vi "EPTxRTmul-inj_Timing1.0.vi"(3 "Control_Config_in":T13={"RT_Input"={"Load"=FALSE, "History_[CAD]"=63, "Stall_Speed_[RPM]"=200.0, "Delay_time[ms]"=0.0}, " PatternConfig"={"Aux_Offset_1_[CAD]"=0.0, "Aux_Offset_2_[CAD]"=0.0, "Aux_Offset_3_[CAD]"=0.0, "Aux_Offset_4_[CAD]"=0.0, "Max_Rate_[Hz]"=0.0}, "SimulatorConfig"={"Sim_Speed_[RPM]"=1000.0, "Ramp_Rate"=50.0, "Rotations"=2, "Pause"=FALSE, "Pause_Angle_[CAD]"=0.0, "Max_Offset_[RPM]"=0.0, "Cylinders"=6}, "EPTxState"={"Sync_Enable"=TRUE, "Clear_Errors"=FALSE, "Sim_Enable"=FALSE, "Sim_Speed_[RPM]"=1000.0}, "EPTxFilters"={"Primary_[s]"=5e-06, "Aux_1_[s]"=5e-06, "Aux_2_[s]"=0.0, "Aux_3_[s]"=0.0, "Aux_4_[s]"=0.0}, "EPTxSupervisor_rt"={"Sync"=FALSE, "CurrentCAD"=0.0, "MaxCAD"=720.0, "HistoryCAD"=61.0, "CADRate"=0.0, "AvgSpeed"=0.0, "Config"=FALSE, "Rcvg_Primary"=FALSE, "Stall"=FALSE, "Overflow"=FALSE, "Ratio_Error"=FALSE, "Pattern_Error"=FALSE, "Aux_Warning"=FALSE, "Watchdog_Error"=FALSE}, "Control_strategy_input"={"Injection_DBTDC"=6.0, "Injection_duration[ms]"=2.0}} caption="簇" {"EPTxFilters"."Aux_4_[s]" format="%#_6p"; "EPTxFilters"."Aux_3_[s]" format="%#_6p"; "EPTxFilters"."Aux_2_[s]" format="%#_6p"; "EPTxFilters"."Aux_1_[s]" format="%#_6p"; "EPTxFilters"."Primary_[s]" format="%#_6p"; "PatternConfig"."Max_Rate_[Hz]" format="%#_3p"}) -> (0 "Control_Config_out":T7={"Config_number"={"EPTxConfig"=0, "EPTxSimulatorConfig"=0}, "Lighting"={"Pattern_Loading"=FALSE, "Sim_Loading"=FALSE, "Config_Loading"=FALSE}, "CylinderSig"={"CylinderSig_1"={"Cylinder1_H_R[CAD]"=204.0, "Cylinder1_H_F[CAD]"=210.0}, "CylinderSig_2"={"Cylinder2_H_R[CAD]"=684.0, "Cylinder2_H_F[CAD]"=690.0}, "CylinderSig_3"={"Cylinder3_H_R[CAD]"=444.0, "Cylinder3_H_F[CAD]"=450.0}, "CylinderSig_4"={"Cylinder4_H_R[CAD]"=90.0, "Cylinder4_H_F[CAD]"=100.0}, "CylinderSig_5"={"Cylinder5_H_R[CAD]"=324.0, "Cylinder5_H_F[CAD]"=330.0}, "CylinderSig_6"={"Cylinder6_H_R[CAD]"=0.0, "Cylinder6_H_F[CAD]"=0.0}}, "EPTxPatternConfig"={"Address"=0.0, "Pattern"={"Primary"=0.0, "Primary_State"=FALSE, "Aux_1"=0.0, "Aux_1_State"=FALSE, "Aux_2"=0.0, "Aux_2_State"=FALSE, "Aux_3"=0.0, "Aux_3_State"=FALSE, "Aux_4"=0.0, "Aux_4_State"=FALSE}}, "EPTxControl"={"Sync_Enable"=FALSE, "Clear_Errors"=FALSE, "Sim_Enable"=FALSE, "Sim_Rate"=63.999996185302734, "Watchdog"=FALSE}, "Tick_output"={"Duration[Ticks]"=0, "Delay[Ticks]"=0}, "EPTxData"={"Sync"=TRUE, "CurrentCAD"=122.91406, "Speed_[RPM]"=999.75, "Config"=FALSE, "Rcvg_Primary"=TRUE, "Stall"=FALSE, "Overflow"=FALSE, "Ratio_Error"=FALSE, "Pattern_Error"=FALSE, "Aux_Warning"=FALSE, "Watchdog_Error"=FALSE}} caption="簇" {"EPTxPatternConfig"."Pattern"."Aux_4" format="%#_16g"; "EPTxPatternConfig"."Pattern"."Aux_3" format="%#_16g"; "EPTxPatternConfig"."Pattern"."Aux_2" format="%#_16g"; "EPTxPatternConfig"."Pattern"."Aux_1" format="%#_16g"; "EPTxPatternConfig"."Pattern"."Primary" format="%#_16g"})   [LabVIEW 2020]
uses:
  <vilib>/Powertrain Controls/Device Drivers/Engine Position Tracking/EPTx/RevA/RT/Controls/Pattern Config.ctl
  <vilib>/Powertrain Controls/Device Drivers/Engine Position Tracking/EPTx/RevA/RT/Controls/Simulator Config.ctl
  <vilib>/Powertrain Controls/Device Drivers/Engine Position Tracking/EPTx/RevA/RT/Controls/EPTxState.ctl
  <vilib>/Powertrain Controls/Device Drivers/Engine Position Tracking/EPTx/RevA/RT/Controls/EPTxFilters.ctl
  <vilib>/Powertrain Controls/Device Drivers/Engine Position Tracking/EPTx/RevA/FPGA/Controls/EPTxSupervisor.ctl
  <vilib>/Powertrain Controls/Device Drivers/Engine Position Tracking/EPTx/RevA/FPGA/Controls/EPTxConfig.ctl
  <vilib>/Powertrain Controls/Device Drivers/Engine Position Tracking/EPTx/RevA/FPGA/Controls/EPTxSimulatorConfig.ctl
  <vilib>/Powertrain Controls/Device Drivers/Engine Position Tracking/EPTx/RevA/FPGA/Controls/EPTxPatternConfig.ctl
  <vilib>/Powertrain Controls/Device Drivers/Engine Position Tracking/EPTx/RevA/FPGA/Controls/Patterns.ctl
  <vilib>/Powertrain Controls/Device Drivers/Engine Position Tracking/EPTx/RevA/FPGA/Controls/EPTxControl.ctl
  <vilib>/Powertrain Controls/Device Drivers/Engine Position Tracking/EPTx/RevA/RT/Controls/EPTxData.ctl
  <vilib>/Powertrain Controls/Device Drivers/Engine Position Tracking/EPTx/RevA/RT/Controls/EPTxPattern.ctl
  <vilib>/Powertrain Controls/Device Drivers/Engine Position Tracking/EPTx/RevA/RT/Controls/Pattern.ctl
  <vilib>/Powertrain Controls/Device Drivers/Engine Position Tracking/EPTx/RevA/RT/Controls/EPTxSettings.ctl
  <vilib>/Powertrain Controls/Device Drivers/Engine Position Tracking/EPTx/RevA/RT/Controls/Settings - Tooth.ctl
  <vilib>/Powertrain Controls/Device Drivers/Engine Position Tracking/EPTx/RevA/RT/Controls/Direction Detection.ctl
  <vilib>/Powertrain Controls/Device Drivers/Engine Position Tracking/EPTx/RevA/RT/Controls/Settings - Pattern.ctl
  <vilib>/Powertrain Controls/Device Drivers/Engine Position Tracking/EPTx/RevA/RT/Controls/Settings - Token.ctl
  <vilib>/Powertrain Controls/Device Drivers/Engine Position Tracking/EPTx/RevA/RT/Controls/Aux Signal.ctl
  <vilib>/Powertrain Controls/Device Drivers/Engine Position Tracking/EPTx/RevA/RT/Controls/Aux Type.ctl
  <vilib>/Powertrain Controls/Device Drivers/Engine Position Tracking/EPTx/RevA/RT/Controls/Aux Threshold.ctl
  <vilib>/Powertrain Controls/Device Drivers/Engine Position Tracking/EPTx/RevA/RT/EPTx - RevA - RT.lvlib
  <vilib>/Powertrain Controls/Device Drivers/Engine Position Tracking/EPTx/RevA/FPGA/EPTx - RevA - FPGA.lvlib
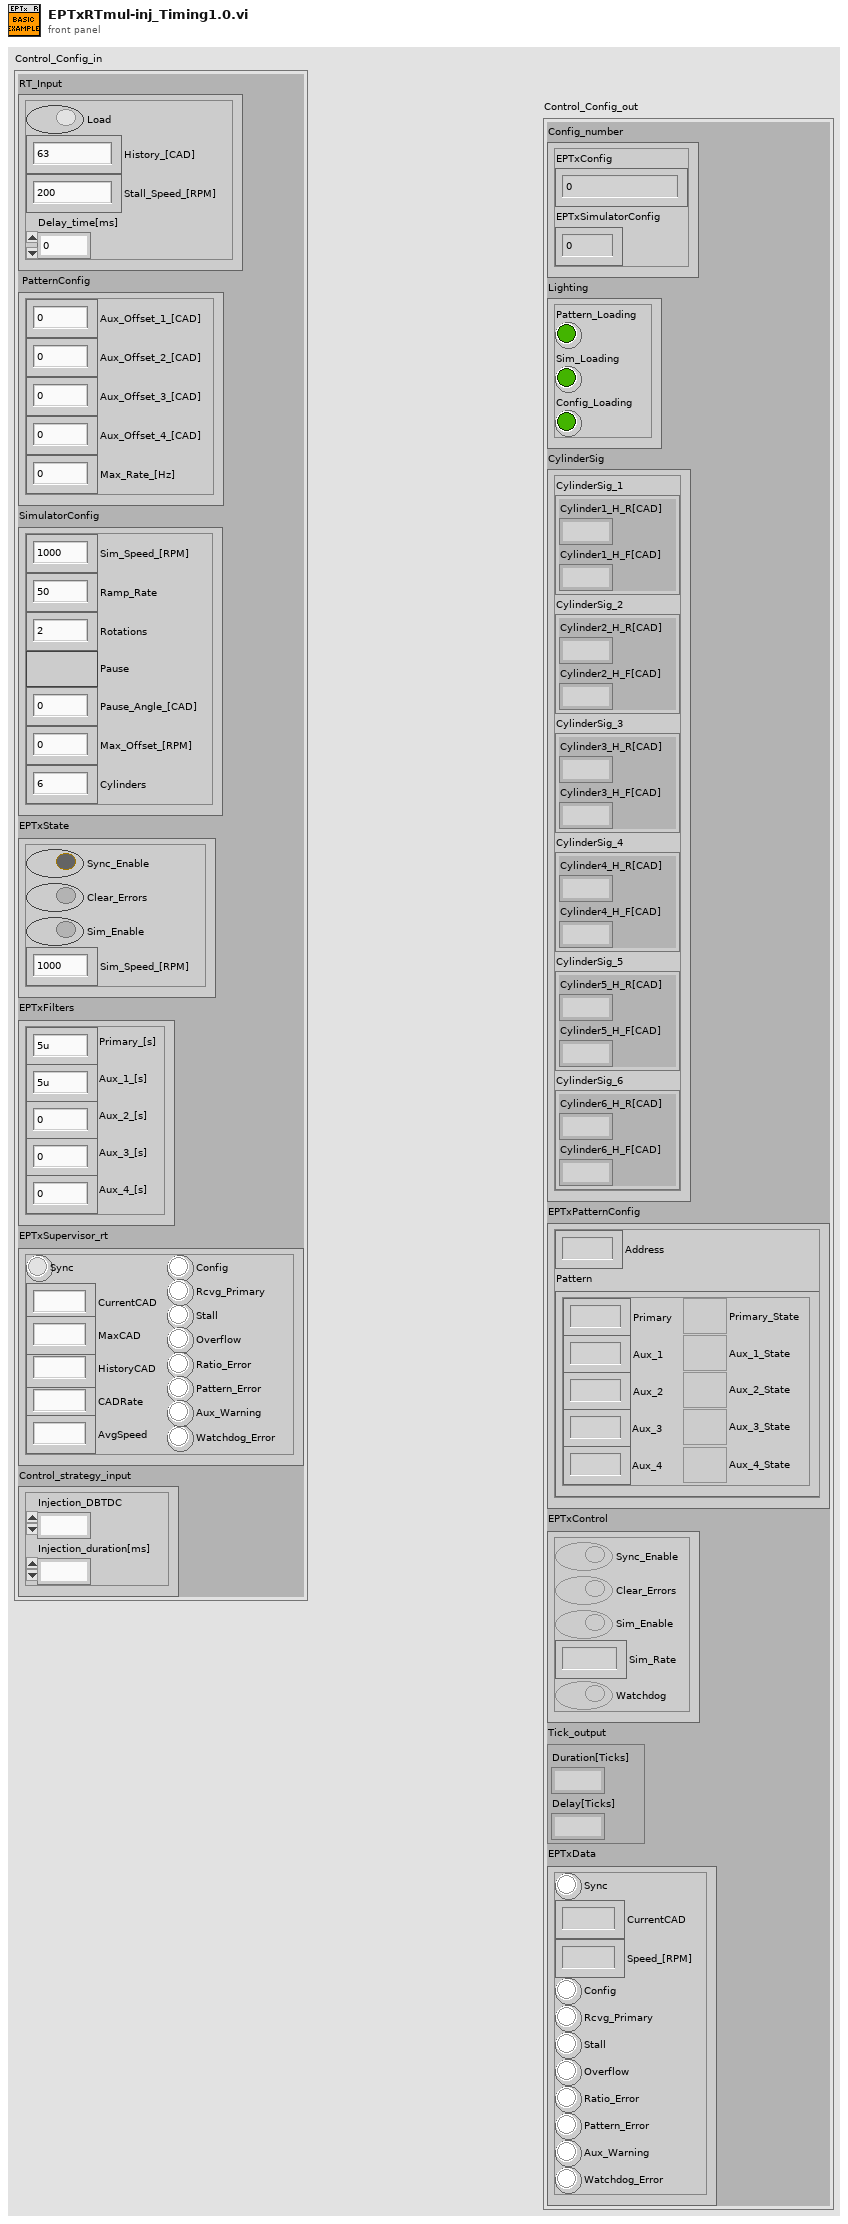
[diagram p1: front panel]
types:
  T1 = typedef "EPTx - RevA - FPGA.lvlib/EPTxConfig.ctl" = u64
  T2 = typedef "EPTx - RevA - FPGA.lvlib/EPTxSimulatorConfig.ctl" = u32
  T3 = typedef "EPTx - RevA - FPGA.lvlib/EPTxPatternConfig.ctl" = cluster{"Address":fxp<+,14,14>, "Pattern":T4}
  T4 = typedef "EPTx - RevA - FPGA.lvlib/Patterns.ctl" = cluster{"Primary":fxp<+,19,12>, "Primary_State":bool, "Aux_1":fxp<+,19,12>, "Aux_1_State":bool, "Aux_2":fxp<+,19,12>, "Aux_2_State":bool, "Aux_3":fxp<+,19,12>, "Aux_3_State":bool, "Aux_4":fxp<+,19,12>, "Aux_4_State":bool}
  T5 = typedef "EPTx - RevA - FPGA.lvlib/EPTxControl.ctl" = cluster{"Sync_Enable":bool, "Clear_Errors":bool, "Sim_Enable":bool, "Sim_Rate":fxp<+,24,6>, "Watchdog":bool}
  T6 = typedef "EPTx - RevA - RT.lvlib/EPTxData.ctl" = cluster{"Sync":bool, "CurrentCAD":sgl, "Speed_[RPM]":sgl, "Config":bool, "Rcvg_Primary":bool, "Stall":bool, "Overflow":bool, "Ratio_Error":bool, "Pattern_Error":bool, "Aux_Warning":bool, "Watchdog_Error":bool}
  T7 = cluster{"Config_number":cluster{"EPTxConfig":T1, "EPTxSimulatorConfig":T2}, "Lighting":cluster{"Pattern_Loading":bool, "Sim_Loading":bool, "Config_Loading":bool}, "CylinderSig":cluster{"CylinderSig_1":cluster{"Cylinder1_H_R[CAD]":fxp<+,18,11>, "Cylinder1_H_F[CAD]":fxp<+,18,11>}, "CylinderSig_2":cluster{"Cylinder2_H_R[CAD]":fxp<+,18,11>, "Cylinder2_H_F[CAD]":fxp<+,18,11>}, "CylinderSig_3":cluster{"Cylinder3_H_R[CAD]":fxp<+,18,11>, "Cylinder3_H_F[CAD]":fxp<+,18,11>}, "CylinderSig_4":cluster{"Cylinder4_H_R[CAD]":fxp<+,18,11>, "Cylinder4_H_F[CAD]":fxp<+,18,11>}, "CylinderSig_5":cluster{"Cylinder5_H_R[CAD]":fxp<+,18,11>, "Cylinder5_H_F[CAD]":fxp<+,18,11>}, "CylinderSig_6":cluster{"Cylinder6_H_R[CAD]":fxp<+,18,11>, "Cylinder6_H_F[CAD]":fxp<+,18,11>}}, "EPTxPatternConfig":T3, "EPTxControl":T5, "Tick_output":cluster{"Duration[Ticks]":u16, "Delay[Ticks]":u16}, "EPTxData":T6}
  T8 = typedef "EPTx - RevA - RT.lvlib/Pattern Config.ctl" = cluster{"Aux_Offset_1_[CAD]":sgl, "Aux_Offset_2_[CAD]":sgl, "Aux_Offset_3_[CAD]":sgl, "Aux_Offset_4_[CAD]":sgl, "Max_Rate_[Hz]":sgl}
  T9 = typedef "EPTx - RevA - RT.lvlib/Simulator Config.ctl" = cluster{"Sim_Speed_[RPM]":sgl, "Ramp_Rate":sgl, "Rotations":u8, "Pause":bool, "Pause_Angle_[CAD]":sgl, "Max_Offset_[RPM]":sgl, "Cylinders":u8}
  T10 = typedef "EPTx - RevA - RT.lvlib/EPTxState.ctl" = cluster{"Sync_Enable":bool, "Clear_Errors":bool, "Sim_Enable":bool, "Sim_Speed_[RPM]":sgl}
  T11 = typedef "EPTx - RevA - RT.lvlib/EPTxFilters.ctl" = cluster{"Primary_[s]":sgl, "Aux_1_[s]":sgl, "Aux_2_[s]":sgl, "Aux_3_[s]":sgl, "Aux_4_[s]":sgl}
  T12 = typedef "EPTx - RevA - FPGA.lvlib/EPTxSupervisor.ctl" = cluster{"Sync":bool, "CurrentCAD":fxp<+,18,11>, "MaxCAD":fxp<+,11,11>, "HistoryCAD":fxp<+,11,11>, "CADRate":fxp<+,22,8>, "AvgSpeed":fxp<+,17,15>, "Config":bool, "Rcvg_Primary":bool, "Stall":bool, "Overflow":bool, "Ratio_Error":bool, "Pattern_Error":bool, "Aux_Warning":bool, "Watchdog_Error":bool}
  T13 = cluster{"RT_Input":cluster{"Load":bool, "History_[CAD]":u8, "Stall_Speed_[RPM]":sgl, "Delay_time[ms]":sgl}, " PatternConfig":T8, "SimulatorConfig":T9, "EPTxState":T10, "EPTxFilters":T11, "EPTxSupervisor_rt":T12, "Control_strategy_input":cluster{"Injection_DBTDC":sgl, "Injection_duration[ms]":sgl}}
  T14 = cluster{"Duration[Ticks]":u16, "Delay[Ticks]":u16}
  T15 = cluster{"CylinderSig_1":cluster{"Cylinder1_H_R [CAD]":fxp<+,18,11>, "Cylinder1_H_F [CAD]":fxp<+,18,11>}, "CylinderSig_2":cluster{"Cylinder2_H_R [CAD]":fxp<+,18,11>, "Cylinder2_H_F [CAD]":fxp<+,18,11>}, "CylinderSig_3":cluster{"Cylinder3_H_R [CAD]":fxp<+,18,11>, "Cylinder3_H_F [CAD]":fxp<+,18,11>}, "CylinderSig_4":cluster{"Cylinder4_H_R [CAD]":fxp<+,18,11>, "Cylinder4_H_F [CAD]":fxp<+,18,11>}, "CylinderSig_5":cluster{"Cylinder5_H_R [CAD]":fxp<+,18,11>, "Cylinder5_H_F [CAD]":fxp<+,18,11>}, "CylinderSig_6":cluster{"Cylinder6_H_R [CAD]":fxp<+,18,11>, "Cylinder6_H_F [CAD]":fxp<+,18,11>}}
  T16 = cluster{"Cylinder6_H_R [CAD]":fxp<+,18,11>, "Cylinder6_H_F [CAD]":fxp<+,18,11>}
  T17 = cluster{"Cylinder5_H_R [CAD]":fxp<+,18,11>, "Cylinder5_H_F [CAD]":fxp<+,18,11>}
  T18 = cluster{"Cylinder4_H_R [CAD]":fxp<+,18,11>, "Cylinder4_H_F [CAD]":fxp<+,18,11>}
  T19 = cluster{"Cylinder3_H_R [CAD]":fxp<+,18,11>, "Cylinder3_H_F [CAD]":fxp<+,18,11>}
  T20 = cluster{"Cylinder2_H_R [CAD]":fxp<+,18,11>, "Cylinder2_H_F [CAD]":fxp<+,18,11>}
  T21 = cluster{"Cylinder1_H_R [CAD]":fxp<+,18,11>, "Cylinder1_H_F [CAD]":fxp<+,18,11>}
  T22 = cluster{"EPTxConfig":T1, "EPTxSimulatorConfig":T2}
  T23 = cluster{"Pattern Loading":bool, "Sim Loading":bool, "Config Loading":bool}
  T24 = cluster{"Load":bool, "History_[CAD]":u8, "Stall_Speed_[RPM]":sgl, "Delay_time[ms]":sgl}
  T25 = cluster{"Injection_DBTDC":sgl, "Injection_duration[ms]":sgl}
  T26 = typedef "EPTx - RevA - RT.lvlib/EPTxSettings.ctl" = cluster{"Rotation":u8, "Ratios":sgl[], "Thresholds":sgl[], "Tooth":T27, "Pattern":T29[], "Token":T30[], "Aux Threshold Min":T33, "Aux Threshold Max":T33}
  T27 = typedef "EPTx - RevA - RT.lvlib/Settings - Tooth.ctl" = cluster{"Rising Edge":bool, "Falling Edge":bool, "Direction\nDetection":T28, "Level":bool, "Parameter":sgl}
  T28 = typedef "EPTx - RevA - RT.lvlib/Direction Detection.ctl" = enum16{"None", "Aux Signal", "Length"}
  T29 = typedef "EPTx - RevA - RT.lvlib/Settings - Pattern.ctl" = cluster{"Ratio Index":u8, "Ratio Count":u16, "Angle":sgl, "dAngle":sgl}
  T30 = typedef "EPTx - RevA - RT.lvlib/Settings - Token.ctl" = cluster{"Length":u16, "Start Index":u8, "Start Count":u16, "Aux 1":T31, "Aux 1 Type":T32, "Aux 1 Max":u16, "Aux 1 Min":u16, "Aux 2":T31, "Aux 2 Type":T32, "Aux 2 Max":u16, "Aux 2 Min":u16, "End Index":u8, "End Count":u16}
  T31 = typedef "EPTx - RevA - RT.lvlib/Aux Signal.ctl" = enum8{"---", "Aux 1", "Aux 2", "Aux 3", "Aux 4"}
  T32 = typedef "EPTx - RevA - RT.lvlib/Aux Type.ctl" = enum8{"Falling", "Rising", "Low", "High", "Ratio"}
  T33 = typedef "EPTx - RevA - RT.lvlib/Aux Threshold.ctl" = cluster{"Aux 1":sgl, "Aux 2":sgl, "Aux 3":sgl, "Aux 4":sgl}
  T34 = typedef "EPTx - RevA - RT.lvlib/EPTxPattern.ctl" = cluster{"Rotations":u8, "Cylinders":u8, "Primary":T35[], "Aux 1":T35[], "Aux 2":T35[], "Aux 3":T35[], "Aux 4":T35[]}
  T35 = typedef "EPTx - RevA - RT.lvlib/Pattern.ctl" = cluster{"Angle":sgl, "State":bool}
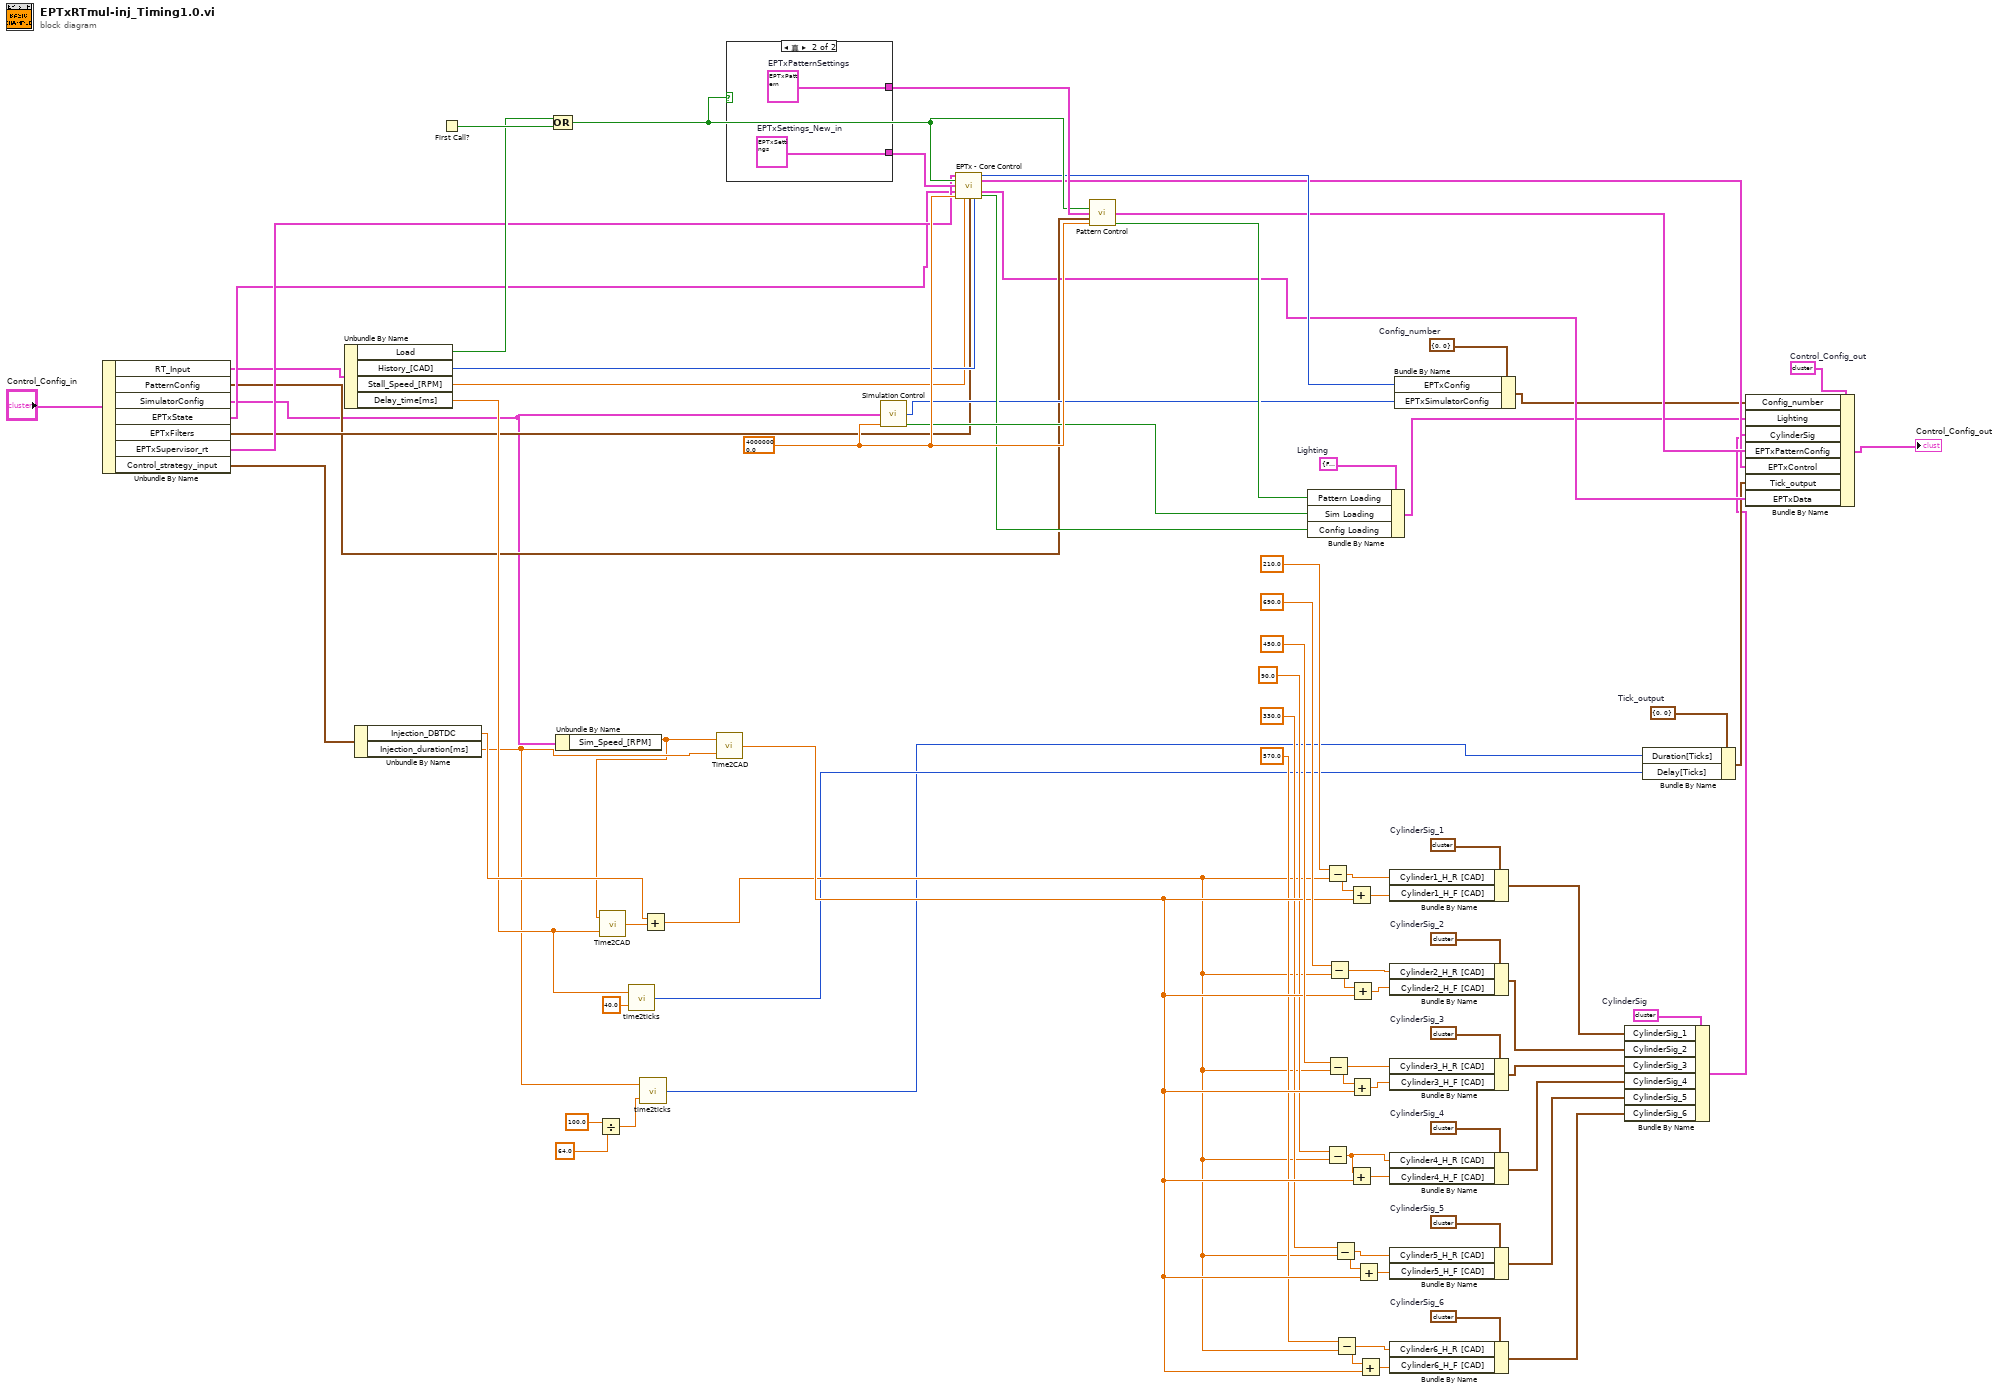
[diagram p0: block diagram]
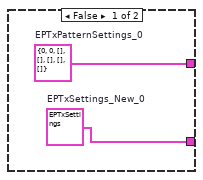
[diagram p2: hidden frame]
diagram:
  w10 = T7 {"Config_number"={"EPTxConfig"=0, "EPTxSimulatorConfig"=0}, "Lighting"={"Pattern_Loading"=FALSE, "Sim_Loading"=FALSE, "Config_Loading"=FALSE}, "CylinderSig"={"CylinderSig_1"={"Cylinder1_H_R[CAD]"=204.0, "Cylinder1_H_F[CAD]"=210.0}, "CylinderSig_2"={"Cylinder2_H_R[CAD]"=684.0, "Cylinder2_H_F[CAD]"=690.0}, "CylinderSig_3"={"Cylinder3_H_R[CAD]"=444.0, "Cylinder3_H_F[CAD]"=450.0}, "CylinderSig_4"={"Cylinder4_H_R[CAD]"=90.0, "Cylinder4_H_F[CAD]"=100.0}, "CylinderSig_5"={"Cylinder5_H_R[CAD]"=324.0, "Cylinder5_H_F[CAD]"=330.0}, "CylinderSig_6"={"Cylinder6_H_R[CAD]"=0.0, "Cylinder6_H_F[CAD]"=0.0}}, "EPTxPatternConfig"={"Address"=0.0, "Pattern"={"Primary"=0.0, "Primary_State"=FALSE, "Aux_1"=0.0, "Aux_1_State"=FALSE, "Aux_2"=0.0, "Aux_2_State"=FALSE, "Aux_3"=0.0, "Aux_3_State"=FALSE, "Aux_4"=0.0, "Aux_4_State"=FALSE}}, "EPTxControl"={"Sync_Enable"=FALSE, "Clear_Errors"=FALSE, "Sim_Enable"=FALSE, "Sim_Rate"=63.999996185302734, "Watchdog"=FALSE}, "Tick_output"={"Duration[Ticks]"=0, "Delay[Ticks]"=0}, "EPTxData"={"Sync"=TRUE, "CurrentCAD"=122.91406, "Speed_[RPM]"=999.75, "Config"=FALSE, "Rcvg_Primary"=TRUE, "Stall"=FALSE, "Overflow"=FALSE, "Ratio_Error"=FALSE, "Pattern_Error"=FALSE, "Aux_Warning"=FALSE, "Watchdog_Error"=FALSE}}  # Control_Config_out
  w25 = T14 {"Duration[Ticks]"=0, "Delay[Ticks]"=0}  # Tick_output
  w41 = T15 {"CylinderSig_1"={"Cylinder1_H_R [CAD]"=204.0, "Cylinder1_H_F [CAD]"=210.0}, "CylinderSig_2"={"Cylinder2_H_R [CAD]"=684.0, "Cylinder2_H_F [CAD]"=690.0}, "CylinderSig_3"={"Cylinder3_H_R [CAD]"=444.0, "Cylinder3_H_F [CAD]"=450.0}, "CylinderSig_4"={"Cylinder4_H_R [CAD]"=90.0, "Cylinder4_H_F [CAD]"=100.0}, "CylinderSig_5"={"Cylinder5_H_R [CAD]"=324.0, "Cylinder5_H_F [CAD]"=330.0}, "CylinderSig_6"={"Cylinder6_H_R [CAD]"=0.0, "Cylinder6_H_F [CAD]"=0.0}}  # CylinderSig
  w58 = T16 {"Cylinder6_H_R [CAD]"=0.0, "Cylinder6_H_F [CAD]"=0.0}  # CylinderSig_6
  w59 = T17 {"Cylinder5_H_R [CAD]"=324.0, "Cylinder5_H_F [CAD]"=330.0}  # CylinderSig_5
  w60 = T18 {"Cylinder4_H_R [CAD]"=90.0, "Cylinder4_H_F [CAD]"=100.0}  # CylinderSig_4
  w61 = T19 {"Cylinder3_H_R [CAD]"=444.0, "Cylinder3_H_F [CAD]"=450.0}  # CylinderSig_3
  w62 = T20 {"Cylinder2_H_R [CAD]"=684.0, "Cylinder2_H_F [CAD]"=690.0}  # CylinderSig_2
  w63 = T21 {"Cylinder1_H_R [CAD]"=204.0, "Cylinder1_H_F [CAD]"=210.0}  # CylinderSig_1
  w69 = T22 {"EPTxConfig"=0, "EPTxSimulatorConfig"=0}  # Config_number
  w73 = T23 {"Pattern Loading"=FALSE, "Sim Loading"=FALSE, "Config Loading"=FALSE}  # Lighting
  w77 = sgl 40000000.0 ("Frequency (40M) [Hz]")
  n1 = Unbundle By Name("Control_Config_in") -> ("RT_Input"=w14:T24, "PatternConfig"=w13:T8, "SimulatorConfig"=w12:T9, "EPTxState"=w16:T10, "EPTxFilters"=w15:T11, "EPTxSupervisor_rt"=w17:T12, "Control_strategy_input"=w11:T25)
  n2 = Unbundle By Name(w14) -> ("Load"=w66:bool, "History_[CAD]"=w65:u8, "Stall_Speed_[RPM]"=w64:sgl, "Delay_time[ms]"=w27:sgl)
  n3 = Unbundle By Name(w11) -> ("Injection_DBTDC"=w30:sgl, "Injection_duration[ms]"=w26:sgl)
  n4 = First Call?() -> (First Call?: T/F=w75:bool)
  n5 = Compound Arithmetic op=OR ("复合运算")(w66, w75) -> (w74:bool)
  n6 = Unbundle By Name(w12) -> ("Sim_Speed_[RPM]"=w1:sgl)
  n7 = Divide(x=100.0, y=64.0) -> (x/y=w19:dbl)
  n8 = call <vilib>:"Time2CAD.vi"("Time [ms]"=w27, "Speed (RPM)"=w1) -> ("CAD"=w28:sgl)
  n9 = call <vilib>:"time2ticks.vi"("Clock Frequency (MHz, 40)"=sgl 40.0, "Time (msec)"=w27) -> ("Ticks"=w24:u32)
  n10 = call <vilib>:"time2ticks.vi"("Clock Frequency (MHz, 40)"=w19, "Time (msec)"=w26) -> ("Ticks"=w23:u32)
  n11 = Add(x=w30, y=w28) -> (x+y=w29:sgl)
  n12 = call <vilib>:"Time2CAD.vi"("Time [ms]"=w26, "Speed (RPM)"=w1) -> ("CAD"=w45:sgl)
  n13 = case shown="真" w74 {
    tunnel: [w79 w81] -> w76
    tunnel: [w78 w80] -> w31
    frame False {
      w78 = T26 {"Rotation"=0, "Ratios"=[], "Thresholds"=[], "Tooth"={"Rising Edge"=FALSE, "Falling Edge"=FALSE, "Direction\nDetection"=enum."None", "Level"=FALSE, "Parameter"=0.0}, "Pattern"=[], "Token"=[], "Aux Threshold Min"={"Aux 1"=0.0, "Aux 2"=0.0, "Aux 3"=0.0, "Aux 4"=0.0}, "Aux Threshold Max"={"Aux 1"=0.0, "Aux 2"=0.0, "Aux 3"=0.0, "Aux 4"=0.0}}  # EPTxSettings_New_0
      w79 = T34 {"Rotations"=0, "Cylinders"=0, "Primary"=[], "Aux 1"=[], "Aux 2"=[], "Aux 3"=[], "Aux 4"=[]}  # EPTxPatternSettings_0
    }
    frame True {
      w80 = T26 {"Rotation"=2, "Ratios"=[0.33333334, 1.0, 3.0], "Thresholds"=[0.16666667, 0.6666667, 0.6666667, 2.0, 2.0, 4.0, 999.0], "Tooth"={"Rising Edge"=TRUE, "Falling Edge"=FALSE, "Direction\nDetection"=enum."None", "Level"=FALSE, "Parameter"=0.0}, "Pattern"=[{"Ratio Index"=0, "Ratio Count"=1, "Angle"=0.0, "dAngle"=6.0}, {"Ratio Index"=1, "Ratio Count"=56, "Angle"=6.0, "dAngle"=6.0}, {"Ratio Index"=2, "Ratio Count"=1, "Angle"=342.0, "dAngle"=18.0}, {"Ratio Index"=0, "Ratio Count"=1, "Angle"=360.0, "dAngle"=6.0}, {"Ratio Index"=1, "Ratio Count"=56, "Angle"=366.0, "dAngle"=6.0}, {"Ratio Index"=2, "Ratio Count"=1, "Angle"=702.0, "dAngle"=18.0}], "Token"=[{"Length"=1, "Start Index"=5, "Start Count"=0, "Aux 1"=enum."---", "Aux 1 Type"=enum."Falling", "Aux 1 Max"=0, "Aux 1 Min"=0, "Aux 2"=enum."Aux 2", "Aux 2 Type"=enum."Ratio", "Aux 2 Max"=73, "Aux 2 Min"=73, "End Index"=0, "End Count"=0}], "Aux Threshold Min"={"Aux 1"=1.8809524, "Aux 2"=1.2142857, "Aux 3"=0.0, "Aux 4"=0.0}, "Aux Threshold Max"={"Aux 1"=2.7857144, "Aux 2"=1.8809524, "Aux 3"=999.0, "Aux 4"=999.0}}  # EPTxSettings_New_in
      w81 = T34 {"Rotations"=2, "Cylinders"=6, "Primary"=[{"Angle"=0.0, "State"=FALSE}, {"Angle"=3.0, "State"=TRUE}, {"Angle"=6.0, "State"=FALSE}, {"Angle"=9.0, "State"=TRUE}, {"Angle"=12.0, "State"=FALSE}, {"Angle"=15.0, "State"=TRUE}, {"Angle"=18.0, "State"=FALSE}, {"Angle"=21.0, "State"=TRUE}, {"Angle"=24.0, "State"=FALSE}, {"Angle"=27.0, "State"=TRUE}, {"Angle"=30.0, "State"=FALSE}, {"Angle"=33.0, "State"=TRUE}, {"Angle"=36.0, "State"=FALSE}, {"Angle"=39.0, "State"=TRUE}, {"Angle"=42.0, "State"=FALSE}, {"Angle"=45.0, "State"=TRUE}, {"Angle"=48.0, "State"=FALSE}, {"Angle"=51.0, "State"=TRUE}, {"Angle"=54.0, "State"=FALSE}, {"Angle"=57.0, "State"=TRUE}, {"Angle"=60.0, "State"=FALSE}, {"Angle"=63.0, "State"=TRUE}, {"Angle"=66.0, "State"=FALSE}, {"Angle"=69.0, "State"=TRUE}, {"Angle"=72.0, "State"=FALSE}, {"Angle"=75.0, "State"=TRUE}, {"Angle"=78.0, "State"=FALSE}, {"Angle"=81.0, "State"=TRUE}, {"Angle"=84.0, "State"=FALSE}, {"Angle"=87.0, "State"=TRUE}, {"Angle"=90.0, "State"=FALSE}, {"Angle"=93.0, "State"=TRUE}, {"Angle"=96.0, "State"=FALSE}, {"Angle"=99.0, "State"=TRUE}, {"Angle"=102.0, "State"=FALSE}, {"Angle"=105.0, "State"=TRUE}, {"Angle"=108.0, "State"=FALSE}, {"Angle"=111.0, "State"=TRUE}, {"Angle"=114.0, "State"=FALSE}, {"Angle"=117.0, "State"=TRUE}, {"Angle"=120.0, "State"=FALSE}, {"Angle"=123.0, "State"=TRUE}, {"Angle"=126.0, "State"=FALSE}, {"Angle"=129.0, "State"=TRUE}, {"Angle"=132.0, "State"=FALSE}, {"Angle"=135.0, "State"=TRUE}, {"Angle"=138.0, "State"=FALSE}, {"Angle"=141.0, "State"=TRUE}, {"Angle"=144.0, "State"=FALSE}, {"Angle"=147.0, "State"=TRUE}, {"Angle"=150.0, "State"=FALSE}, {"Angle"=153.0, "State"=TRUE}, {"Angle"=156.0, "State"=FALSE}, {"Angle"=159.0, "State"=TRUE}, {"Angle"=162.0, "State"=FALSE}, {"Angle"=165.0, "State"=TRUE}, {"Angle"=168.0, "State"=FALSE}, {"Angle"=171.0, "State"=TRUE}, {"Angle"=174.0, "State"=FALSE}, {"Angle"=177.0, "State"=TRUE}, {"Angle"=180.0, "State"=FALSE}, {"Angle"=183.0, "State"=TRUE}, {"Angle"=186.0, "State"=FALSE}, {"Angle"=189.0, "State"=TRUE}, {"Angle"=192.0, "State"=FALSE}, {"Angle"=195.0, "State"=TRUE}, {"Angle"=198.0, "State"=FALSE}, {"Angle"=201.0, "State"=TRUE}, {"Angle"=204.0, "State"=FALSE}, {"Angle"=207.0, "State"=TRUE}, {"Angle"=210.0, "State"=FALSE}, {"Angle"=213.0, "State"=TRUE}, {"Angle"=216.0, "State"=FALSE}, {"Angle"=219.0, "State"=TRUE}, {"Angle"=222.0, "State"=FALSE}, {"Angle"=225.0, "State"=TRUE}, {"Angle"=228.0, "State"=FALSE}, {"Angle"=231.0, "State"=TRUE}, {"Angle"=234.0, "State"=FALSE}, {"Angle"=237.0, "State"=TRUE}, {"Angle"=240.0, "State"=FALSE}, {"Angle"=243.0, "State"=TRUE}, {"Angle"=246.0, "State"=FALSE}, {"Angle"=249.0, "State"=TRUE}, {"Angle"=252.0, "State"=FALSE}, {"Angle"=255.0, "State"=TRUE}, {"Angle"=258.0, "State"=FALSE}, {"Angle"=261.0, "State"=TRUE}, {"Angle"=264.0, "State"=FALSE}, {"Angle"=267.0, "State"=TRUE}, {"Angle"=270.0, "State"=FALSE}, {"Angle"=273.0, "State"=TRUE}, {"Angle"=276.0, "State"=FALSE}, {"Angle"=279.0, "State"=TRUE}, {"Angle"=282.0, "State"=FALSE}, {"Angle"=285.0, "State"=TRUE}, {"Angle"=288.0, "State"=FALSE}, {"Angle"=291.0, "State"=TRUE}, {"Angle"=294.0, "State"=FALSE}, {"Angle"=297.0, "State"=TRUE}, {"Angle"=300.0, "State"=FALSE}, {"Angle"=303.0, "State"=TRUE}, {"Angle"=306.0, "State"=FALSE}, {"Angle"=309.0, "State"=TRUE}, {"Angle"=312.0, "State"=FALSE}, {"Angle"=315.0, "State"=TRUE}, {"Angle"=318.0, "State"=FALSE}, {"Angle"=321.0, "State"=TRUE}, {"Angle"=324.0, "State"=FALSE}, {"Angle"=327.0, "State"=TRUE}, {"Angle"=330.0, "State"=FALSE}, {"Angle"=333.0, "State"=TRUE}, {"Angle"=336.0, "State"=FALSE}, {"Angle"=339.0, "State"=TRUE}, {"Angle"=342.0, "State"=FALSE}, {"Angle"=345.0, "State"=TRUE}, {"Angle"=360.0, "State"=FALSE}, {"Angle"=363.0, "State"=TRUE}, {"Angle"=366.0, "State"=FALSE}, {"Angle"=369.0, "State"=TRUE}, {"Angle"=372.0, "State"=FALSE}, {"Angle"=375.0, "State"=TRUE}, {"Angle"=378.0, "State"=FALSE}, {"Angle"=381.0, "State"=TRUE}, {"Angle"=384.0, "State"=FALSE}, {"Angle"=387.0, "State"=TRUE}, {"Angle"=390.0, "State"=FALSE}, {"Angle"=393.0, "State"=TRUE}, {"Angle"=396.0, "State"=FALSE}, {"Angle"=399.0, "State"=TRUE}, {"Angle"=402.0, "State"=FALSE}, {"Angle"=405.0, "State"=TRUE}, {"Angle"=408.0, "State"=FALSE}, {"Angle"=411.0, "State"=TRUE}, {"Angle"=414.0, "State"=FALSE}, {"Angle"=417.0, "State"=TRUE}, {"Angle"=420.0, "State"=FALSE}, {"Angle"=423.0, "State"=TRUE}, {"Angle"=426.0, "State"=FALSE}, {"Angle"=429.0, "State"=TRUE}, {"Angle"=432.0, "State"=FALSE}, {"Angle"=435.0, "State"=TRUE}, {"Angle"=438.0, "State"=FALSE}, {"Angle"=441.0, "State"=TRUE}, {"Angle"=444.0, "State"=FALSE}, {"Angle"=447.0, "State"=TRUE}, {"Angle"=450.0, "State"=FALSE}, {"Angle"=453.0, "State"=TRUE}, {"Angle"=456.0, "State"=FALSE}, {"Angle"=459.0, "State"=TRUE}, {"Angle"=462.0, "State"=FALSE}, {"Angle"=465.0, "State"=TRUE}, {"Angle"=468.0, "State"=FALSE}, {"Angle"=471.0, "State"=TRUE}, {"Angle"=474.0, "State"=FALSE}, {"Angle"=477.0, "State"=TRUE}, {"Angle"=480.0, "State"=FALSE}, {"Angle"=483.0, "State"=TRUE}, {"Angle"=486.0, "State"=FALSE}, {"Angle"=489.0, "State"=TRUE}, {"Angle"=492.0, "State"=FALSE}, {"Angle"=495.0, "State"=TRUE}, {"Angle"=498.0, "State"=FALSE}, {"Angle"=501.0, "State"=TRUE}, {"Angle"=504.0, "State"=FALSE}, {"Angle"=507.0, "State"=TRUE}, {"Angle"=510.0, "State"=FALSE}, {"Angle"=513.0, "State"=TRUE}, {"Angle"=516.0, "State"=FALSE}, {"Angle"=519.0, "State"=TRUE}, {"Angle"=522.0, "State"=FALSE}, {"Angle"=525.0, "State"=TRUE}, {"Angle"=528.0, "State"=FALSE}, {"Angle"=531.0, "State"=TRUE}, {"Angle"=534.0, "State"=FALSE}, {"Angle"=537.0, "State"=TRUE}, {"Angle"=540.0, "State"=FALSE}, {"Angle"=543.0, "State"=TRUE}, {"Angle"=546.0, "State"=FALSE}, {"Angle"=549.0, "State"=TRUE}, {"Angle"=552.0, "State"=FALSE}, {"Angle"=555.0, "State"=TRUE}, {"Angle"=558.0, "State"=FALSE}, {"Angle"=561.0, "State"=TRUE}, {"Angle"=564.0, "State"=FALSE}, {"Angle"=567.0, "State"=TRUE}, {"Angle"=570.0, "State"=FALSE}, {"Angle"=573.0, "State"=TRUE}, {"Angle"=576.0, "State"=FALSE}, {"Angle"=579.0, "State"=TRUE}, {"Angle"=582.0, "State"=FALSE}, {"Angle"=585.0, "State"=TRUE}, {"Angle"=588.0, "State"=FALSE}, {"Angle"=591.0, "State"=TRUE}, {"Angle"=594.0, "State"=FALSE}, {"Angle"=597.0, "State"=TRUE}, {"Angle"=600.0, "State"=FALSE}, {"Angle"=603.0, "State"=TRUE}, {"Angle"=606.0, "State"=FALSE}, {"Angle"=609.0, "State"=TRUE}, {"Angle"=612.0, "State"=FALSE}, {"Angle"=615.0, "State"=TRUE}, {"Angle"=618.0, "State"=FALSE}, {"Angle"=621.0, "State"=TRUE}, {"Angle"=624.0, "State"=FALSE}, {"Angle"=627.0, "State"=TRUE}, {"Angle"=630.0, "State"=FALSE}, {"Angle"=633.0, "State"=TRUE}, {"Angle"=636.0, "State"=FALSE}, {"Angle"=639.0, "State"=TRUE}, {"Angle"=642.0, "State"=FALSE}, {"Angle"=645.0, "State"=TRUE}, {"Angle"=648.0, "State"=FALSE}, {"Angle"=651.0, "State"=TRUE}, {"Angle"=654.0, "State"=FALSE}, {"Angle"=657.0, "State"=TRUE}, {"Angle"=660.0, "State"=FALSE}, {"Angle"=663.0, "State"=TRUE}, {"Angle"=666.0, "State"=FALSE}, {"Angle"=669.0, "State"=TRUE}, {"Angle"=672.0, "State"=FALSE}, {"Angle"=675.0, "State"=TRUE}, {"Angle"=678.0, "State"=FALSE}, {"Angle"=681.0, "State"=TRUE}, {"Angle"=684.0, "State"=FALSE}, {"Angle"=687.0, "State"=TRUE}, {"Angle"=690.0, "State"=FALSE}, {"Angle"=693.0, "State"=TRUE}, {"Angle"=696.0, "State"=FALSE}, {"Angle"=699.0, "State"=TRUE}, {"Angle"=702.0, "State"=FALSE}, {"Angle"=705.0, "State"=TRUE}], "Aux 1"=[{"Angle"=12.0, "State"=TRUE}, {"Angle"=24.0, "State"=FALSE}, {"Angle"=48.0, "State"=TRUE}, {"Angle"=60.0, "State"=FALSE}, {"Angle"=132.0, "State"=TRUE}, {"Angle"=144.0, "State"=FALSE}, {"Angle"=198.0, "State"=TRUE}, {"Angle"=252.0, "State"=TRUE}, {"Angle"=264.0, "State"=FALSE}, {"Angle"=318.0, "State"=TRUE}, {"Angle"=372.0, "State"=TRUE}, {"Angle"=384.0, "State"=FALSE}, {"Angle"=438.0, "State"=TRUE}, {"Angle"=492.0, "State"=TRUE}, {"Angle"=504.0, "State"=FALSE}, {"Angle"=558.0, "State"=TRUE}, {"Angle"=612.0, "State"=TRUE}, {"Angle"=624.0, "State"=FALSE}, {"Angle"=678.0, "State"=TRUE}], "Aux 2"=[{"Angle"=12.0, "State"=TRUE}, {"Angle"=24.0, "State"=FALSE}, {"Angle"=48.0, "State"=TRUE}, {"Angle"=60.0, "State"=FALSE}, {"Angle"=132.0, "State"=TRUE}, {"Angle"=144.0, "State"=FALSE}, {"Angle"=198.0, "State"=TRUE}, {"Angle"=252.0, "State"=TRUE}, {"Angle"=264.0, "State"=FALSE}, {"Angle"=318.0, "State"=TRUE}, {"Angle"=372.0, "State"=TRUE}, {"Angle"=384.0, "State"=FALSE}, {"Angle"=438.0, "State"=TRUE}, {"Angle"=492.0, "State"=TRUE}, {"Angle"=504.0, "State"=FALSE}, {"Angle"=558.0, "State"=TRUE}, {"Angle"=612.0, "State"=TRUE}, {"Angle"=624.0, "State"=FALSE}, {"Angle"=678.0, "State"=TRUE}], "Aux 3"=[], "Aux 4"=[]}  # EPTxPatternSettings
    }
  }
  n14 = call <vilib>:"Simulation Control.vi"("SimulatorConfig"=w12, "Frequency (40M) [Hz]"=w77) -> ("EPTxSimulatorConfig"=w67:T2, "Loading"=w71:bool)  [unwired: 12 in]
  n15 = call <vilib>:"EPTx - Core Control.vi"("EPTxSupervisor"=w17, "Load"=w74, "EPTxSettings"=w31, "EPTxState"=w16, "Frequency (40M) [Hz]"=w77, "Stall Speed (200) [RPM]"=w64, "Filters (0)"=w15, "History (63) [CAD]"=w65) -> ("EPTxConfig"=w68:T1, "EPTxControl"=w8:T5, "EPTxData"=w7:T6, "Loading"=w70:bool)  [unwired: 3 in, 1 out]
  n16 = call <vilib>:"Pattern Control.vi"("Load"=w74, "EPTxPatternSettings"=w76, "PatternConfig"=w13, "Frequency (40M) [Hz]"=w77) -> ("EPTxPatternConfig"=w9:T3, "Loading"=w72:bool)  [unwired: 10 in]
  n17 = Bundle By Name(cluster=w73, "Pattern Loading"=w72, "Sim Loading"=w71, "Config Loading"=w70) -> (w5:T23)
  n18 = Subtract(x=sgl 210.0 ("Cylinder TDC [Absolute CAD]"), y=w29) -> (x-y=w55:sgl)
  n19 = Subtract(x=sgl 90.0 ("Cylinder TDC [Absolute CAD]"), y=w29) -> (x-y=w32:sgl)
  n20 = Subtract(x=sgl 450.0 ("Cylinder TDC [Absolute CAD]"), y=w29) -> (x-y=w50:sgl)
  n21 = Subtract(x=sgl 690.0 ("Cylinder TDC [Absolute CAD]"), y=w29) -> (x-y=w53:sgl)
  n22 = Subtract(x=sgl 330.0 ("Cylinder TDC [Absolute CAD]"), y=w29) -> (x-y=w33:sgl)
  n23 = Subtract(x=sgl 570.0 ("Cylinder TDC [Absolute CAD]"), y=w29) -> (x-y=w34:sgl)
  n24 = Add(x=w55, y=w45) -> (x+y=w56:sgl)
  n25 = Add(x=w32, y=w45) -> (x+y=w48:sgl)
  n26 = Add(x=w50, y=w45) -> (x+y=w51:sgl)
  n27 = Add(x=w53, y=w45) -> (x+y=w54:sgl)
  n28 = Add(x=w33, y=w45) -> (x+y=w47:sgl)
  n29 = Add(x=w34, y=w45) -> (x+y=w46:sgl)
  n30 = Bundle By Name(cluster=w63, "Cylinder1_H_R [CAD]"=w55, "Cylinder1_H_F [CAD]"=w56) -> (w40:T21)
  n31 = Bundle By Name(cluster=w62, "Cylinder2_H_R [CAD]"=w53, "Cylinder2_H_F [CAD]"=w54) -> (w39:T20)
  n32 = Bundle By Name(cluster=w61, "Cylinder3_H_R [CAD]"=w50, "Cylinder3_H_F [CAD]"=w51) -> (w38:T19)
  n33 = Bundle By Name(cluster=w60, "Cylinder4_H_R [CAD]"=w32, "Cylinder4_H_F [CAD]"=w48) -> (w37:T18)
  n34 = Bundle By Name(cluster=w59, "Cylinder5_H_R [CAD]"=w33, "Cylinder5_H_F [CAD]"=w47) -> (w36:T17)
  n35 = Bundle By Name(cluster=w58, "Cylinder6_H_R [CAD]"=w34, "Cylinder6_H_F [CAD]"=w46) -> (w35:T16)
  n36 = Bundle By Name(cluster=w69, "EPTxConfig"=w68, "EPTxSimulatorConfig"=w67) -> (w6:T22)
  n37 = Bundle By Name(cluster=w41, "CylinderSig_1"=w40, "CylinderSig_2"=w39, "CylinderSig_3"=w38, "CylinderSig_4"=w37, "CylinderSig_5"=w36, "CylinderSig_6"=w35) -> (w2:T15)
  n38 = Bundle By Name(cluster=w25, "Duration[Ticks]"=w23, "Delay[Ticks]"=w24) -> (w3:T14)
  n39 = Bundle By Name(cluster=w10, "Config_number"=w6, "Lighting"=w5, "CylinderSig"=w2, "EPTxPatternConfig"=w9, "EPTxControl"=w8, "Tick_output"=w3, "EPTxData"=w7) -> (→"Control_Config_out":T7)
